vi "Close File.vi"(8 "error in (no error)":errorcluster, 11 "Spectrum Recorder in":refnum<class "Spectrum Recorder too.lvclass">) -> (0 "error out":errorcluster, 2 "Acquired Result.lvclass":refnum<class "Acquired Result.lvclass">, 3 "Spectrum Recorder out":refnum<class "Spectrum Recorder too.lvclass">)   [LabVIEW 2016, in "Spectrum Recorder too.lvclass"]
uses:
  Spectrum Recorder too.lvclass
  C:/github/LabActor/Worker/Worker.lvclass
  NHMFL_Core/Libraries/Instruments/Results/Acquired Result/Acquired Result.lvclass
  NHMFL_Core/Libraries/Instruments/Results/File Path Result/File Path Result.lvclass
  C:/github/NHMFL_Core/Libraries/Instruments/Results/Acquired Result/Acquired Result.lvclass
  Worker/Worker.lvclass/Worker.ctl
  Spectrum Recorder too.lvclass/Spectrum Recorder too.ctl
  NHMFL_Core/Libraries/Instruments/Results/Acquired Result/Acquired Result.lvclass/Acquired Result.ctl
  Worker/Read Cycle count.vi
  Worker/Write Cycle count.vi
  NHMFL_Core/Libraries/Instruments/Results/Acquired Result/Write Cycle count.vi
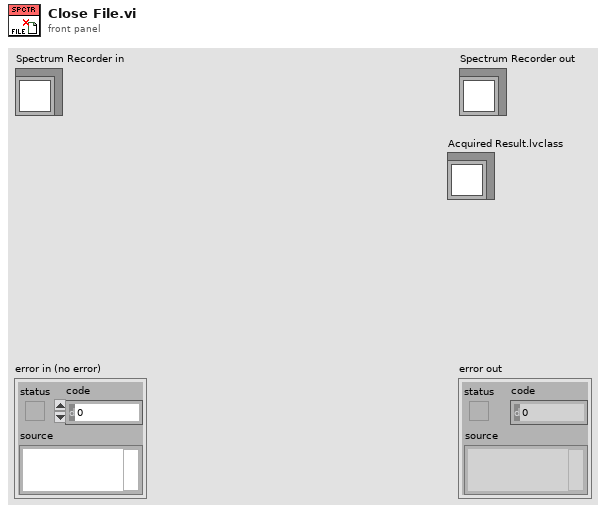
[diagram p1: front panel]
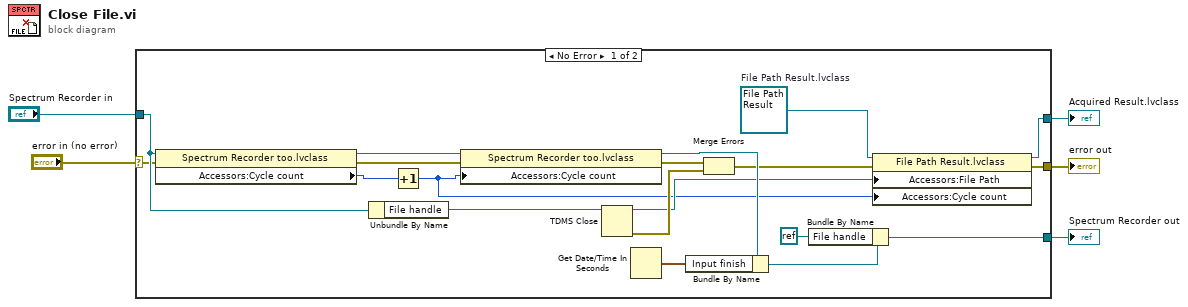
[diagram p0: block diagram]
diagram:
  n1 = case shown="No Error" "error in (no error)" {
    selector: "error in (no error)" -> [w22 w26]
    tunnel: [w17 w26] -> w4
    tunnel: [w23 w25] -> w2
    tunnel: "Spectrum Recorder in" -> [w24 w25]
    tunnel: [w21 _] -> w1
    frame No Error {
      w10 = refnum<class "File Path Result.lvclass"> refnum  # File Path Result.lvclass
      n2 = property class="Spectrum Recorder too.lvclass"(reference=w24, error in=w22) -> (reference out=w16:refnum<class "Spectrum Recorder too.lvclass">, error out=w15:errorcluster, "Accessors:Cycle count"=w14:i32)
      n3 = Unbundle By Name(w24) -> ("File handle"=w20:refnum<k34>)
      n4 = Increment(x=w14) -> (x+1=w6:i32)
      n5 = property class="Spectrum Recorder too.lvclass"(reference=w16, error in=w15, "Accessors:Cycle count"=w6) -> (reference out=w12:refnum<class "Spectrum Recorder too.lvclass">, error out=w13:errorcluster)
      n6 = TDMS Close(11:w20) -> (0:w11:errorcluster, 3:w9:path)  [unwired: 1 in]
      n7 = Get Date/Time In Seconds() -> (seconds since 1Jan1904=w7:timestamp)
      n8 = Bundle By Name(cluster=w12, "Input finish"=w7) -> (w19:refnum<class "Spectrum Recorder too.lvclass">)
      n9 = Merge Errors(w13, w11) -> (w8:errorcluster)
      n10 = Bundle By Name(cluster=w19, "File handle"=refnum<k0> refnum) -> (w23:refnum<class "Spectrum Recorder too.lvclass">)
      n11 = property class="File Path Result.lvclass"(reference=w10, error in=w8, "Accessors:File Path"=w9, "Accessors:Cycle count"=w6) -> (reference out=w21:refnum<class "File Path Result.lvclass">, error out=w17:errorcluster)
    }
    frame Error {
    }
  }
  "error out" <- w4
  "Spectrum Recorder out" <- w2
  "Acquired Result.lvclass" <- w1
